vi "cw_4_10.vi"() -> ()   [LabVIEW 2022 SP3]
panel:
  out "Paliandrom":bool
  in  "String":string
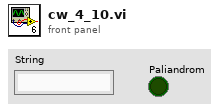
[diagram p1: front panel]
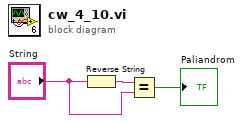
[diagram p0: block diagram]
diagram:
  n1 = Reverse String(1:"String") -> (0:w3:string)
  n2 = Equal?(x=w3, y="String") -> (x = y?=→"Paliandrom":bool)
